vi "test_Create Trigger Message.vi"(8 "error in (no error)":errorcluster, 11 "TestCase in":refnum<class "Instrument Addon Scripting API Messages Unit Tests.lvclass">) -> (0 "error out":errorcluster, 3 "TestCase out":refnum<class "Instrument Addon Scripting API Messages Unit Tests.lvclass">)   [LabVIEW 2018, in "Instrument Addon Scripting API Messages Unit Tests.lvclass"]
uses:
  Instrument Addon Scripting API Messages Unit Tests.lvclass
  NationalInstruments.VeriStand.SystemDefinitionAPI
  APIs/Scripting API/TypeDefs/Message Settings.ctl
  APIs/Scripting API/TypeDefs/Protection Types.ctl
  Addon/Addon Shared/SubVIs/Constants.vi
  <vilib>/NI Veristand/Custom Device Tools/Custom Device Utility Library/NI VeriStand - Search for Item by GUID.vi
  APIs/Scripting API/Messages/Create Message - Trigger Only.vi
  <vilib>/addons/_JKI Toolkits/VI Tester/TestCase.llb/TestCase.lvclass
  Instrument Addon Scripting API Test Assets/Instrument Addon Scripting API Test Assets.lvclass
  APIs/Scripting API/Instrument Addon Scripting API.lvlib
  <vilib>/NI Veristand/Custom Device Tools/Custom Device Utility Library/Custom Device Utility Library.lvlib
  Addon/Addon Shared/Instrument Addon Shared.lvlib
  C:/Program Files (x86)/National Instruments/LabVIEW 2018/vi.lib/addons/_JKI Toolkits/VI Tester/TestCase.llb/TestCase.lvclass
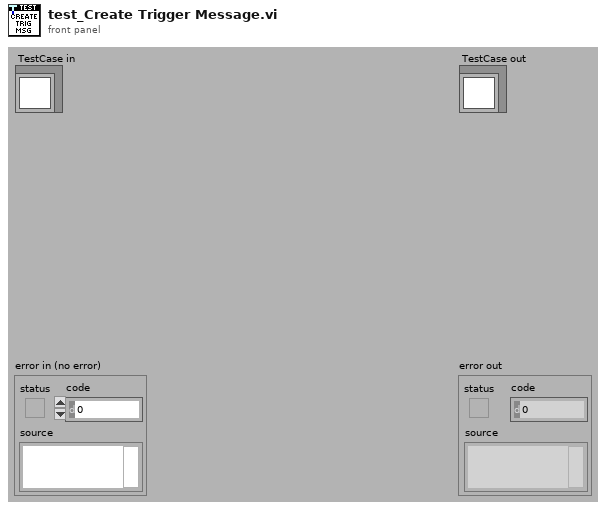
[diagram p1: front panel]
types:
  T1 = typedef "Instrument Addon Scripting API.lvlib/Message Settings.ctl" = cluster{"Protection Types":T2, "Enable Periodic Default":bool, "Trigger Channel Refnum":u64}
  T2 = typedef "Instrument Addon Scripting API.lvlib/Protection Types.ctl" = enum16{"None", "CRC-32", "Checksum U16", "Checksum U32", "Checksum U8"}
  T3 = typedef "Custom Device API.lvlib/Custom Device Item Ref.ctl" = u64
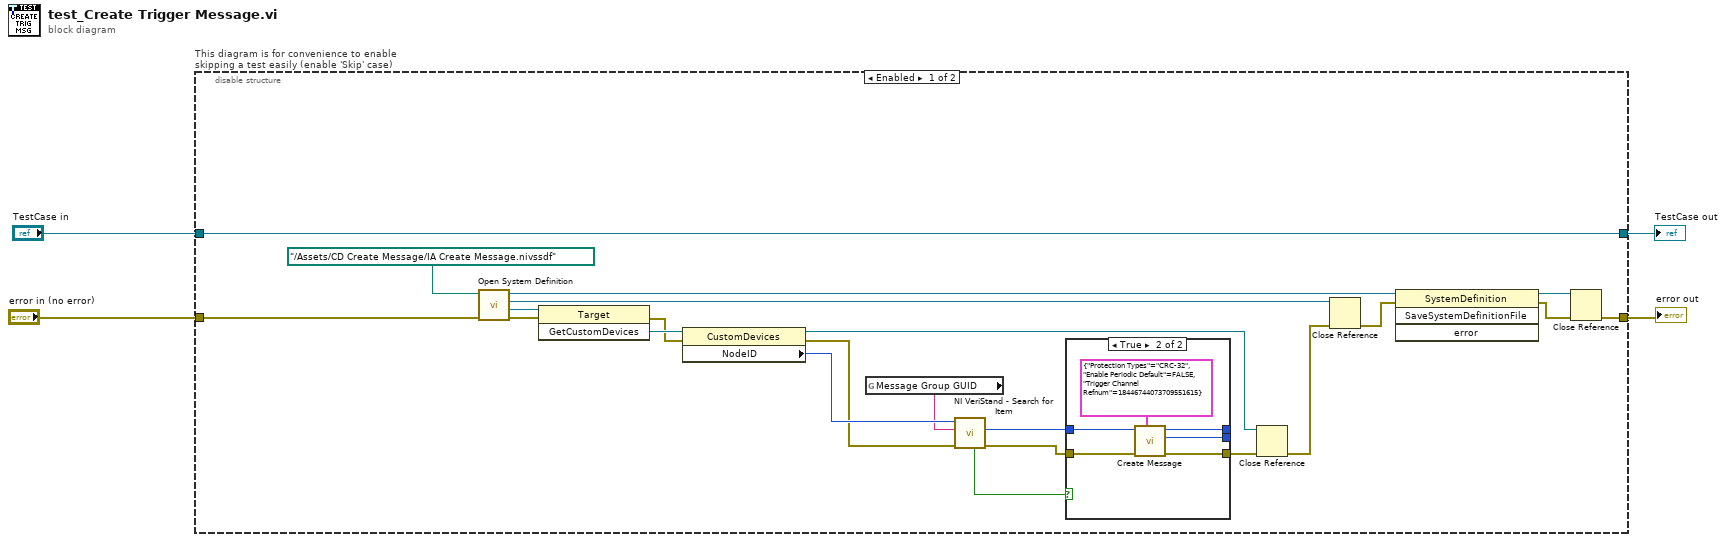
[diagram p0: block diagram]
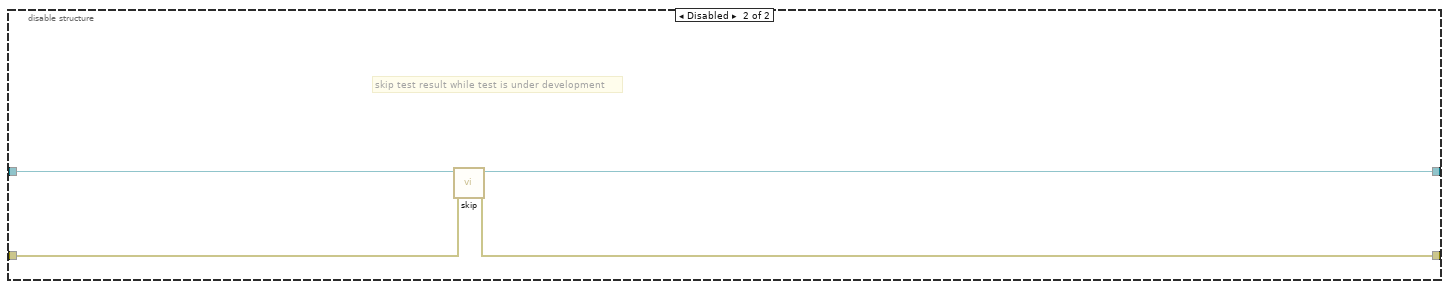
[diagram p3: hidden frame]
diagram:
  n1 = disable-structure "This diagram is for convenience to enable skipping a test easily (enable 'Skip' case)" shown="Enabled" {
    disable-tunnel: "TestCase in" -> [w6 w37]
    disable-tunnel: [w6 w35] -> w1
    disable-tunnel: [w5 w36] -> w3
    disable-tunnel: "error in (no error)" -> [w25 w34]
    frame Enabled {
      n2 = call "Open System Definition.vi"("error in (no error)"=w25, "System Definition File"=path "../Assets/CD Create Message/IA Create Message.nivssdf" ("SDF file")) -> ("error out"=w17:errorcluster, "Target Refnum"=w24:refnum<k24>, "Root Refnum"=w11:refnum<k24>, "System Definition Refnum"=w18:refnum<k24>)  [unwired: 6 in]
      n3 = invoke class="Target" method="GetCustomDevices"(reference=w24, error in=w17) -> (error out=w16:errorcluster, "GetCustomDevices"=w23:refnum<k24>)  [unwired: 1 in, 1 out]
      n4 = property class="CustomDevices"(reference=w23, error in=w16) -> (reference out=w13:refnum<k24>, error out=w15:errorcluster, "NodeID"=w22:u64)
      n5 = global read "Constants.vi" "Message Group GUID"() -> (w21:string)
      n6 = call-poly <vilib>:"NI VeriStand - Search for Item.vi"("error in"=w15, "Item GUID"=w21, "Section Ref in"=w22) -> ("error out"=w14:errorcluster, "Item Ref"=w20:T3, "Found"=w19:bool)  [unwired: 5 in, 1 out]
      n7 = case shown="True" w19 {
        tunnel: w20 -> [_ w33]
        tunnel: [w27 w32] -> w12
        tunnel: w14 -> [w27 w31]
        tunnel: [_ w30] -> _
        tunnel: [_ w29] -> _
        frame False {
        }
        frame True {
          n8 = call-poly "Create Message.vi"("Message Settings"=T1 {"Protection Types"=enum."CRC-32", "Enable Periodic Default"=FALSE, "Trigger Channel Refnum"=18446744073709551615}, "error in (no error)"=w31, "Message Group in"=w33) -> ("error out"=w32:errorcluster, "Message Refnum out"=w30:T3, "Message Goup out"=w29:T3)  [unwired: 6 in]
        }
      }
      n9 = Close Reference(reference=w13, error in (no error)=w12) -> (error out=w10:errorcluster)
      n10 = Close Reference(reference=w11, error in (no error)=w10) -> (error out=w9:errorcluster)
      n11 = invoke class="SystemDefinition" method="SaveSystemDefinitionFile"(reference=w18, error in=w9) -> (reference out=w7:refnum<k24>, error out=w8:errorcluster)  [unwired: 2 in, 2 out]
      n12 = Close Reference(reference=w7, error in (no error)=w8) -> (error out=w5:errorcluster)
    }
    frame Disabled {
      # "skip test result while test is under development"
      n13 = call <vilib>:"skip.vi"("error in (no error)"=w34, "TestCase in"=w37) -> ("error out"=w36:errorcluster, "TestCase out"=w35:refnum<class "Instrument Addon Scripting API Messages Unit Tests.lvclass">)  [unwired: 8 in]
    }
  }
  "error out" <- w3
  "TestCase out" <- w1
